vi "motor.vi"() -> ()   [LabVIEW 2020]
uses:
  <vilib>/High Genius/HG_WSI_Tookit/Dependencies/Library/CAN/CAN.lvclass
  C:/Program Files (x86)/National Instruments/LabVIEW 2020/vi.lib/High Genius/HG_WSI_Tookit/Dependencies/Library/HG_LIB/HG_LIB.lvclass
  <vilib>/Platform/TimedLoop/XDataNode/timing_clust.ctl
  <vilib>/Platform/TimedLoop/XDataNode/nitl_modes.ctl
  <vilib>/Platform/TimedLoop/XDataNode/wakeup.ctl
  <vilib>/platform/TimedLoop/XDataNode/XDataNode.xnode
  <vilib>/High Genius/HG_WSI_Tookit/Dependencies/Library/HG_LIB/HG_LIB.lvclass
  <vilib>/Platform/TimedLoop/XDataNode/XDNodeRunTimeDep.lvlib
panel:
  in  "stop":bool
  in  "Numeric":dbl
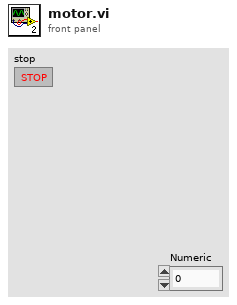
[diagram p1: front panel]
types:
  T1 = enum16{"DI", "DO", "AI", "Pulse", "PWM", "ISQ", "ENC", "CAN", "IIC", "IMU"}
  T2 = enum16{"0", "1", "2", "3", "4", "5", "6", "7", "8", "9", "10", "11", "12", "13", "14", "15", "16", "17", "18", "19", "20", "21", "22", "23", "24", "25"}
  T3 = typedef "XDNodeRunTimeDep.lvlib/timing_clust.ctl" = cluster{"Expected End [f-1]":u64, "Actual End [f-1]":u64, "Finished Late? [f-1]":bool, "Expected End [i-1]":u64, "Actual End [i-1]":u64, "Finished Late? [i-1]":bool, "Expected Start [i]":u64, "Actual Start [i]":u64, "Expected Start [f]":u64, "Actual Start [f]":u64, "Source Name":string, "Structure Name":string, "Period":i64, "Deadline":i64, "Offset":i64, "Start":i64, "Priority":i32, "Timeout":i32, "Mode":T4, "Wakeup Reason":T5, "Error":errorcluster, "Source Type":string, "Secondary Source Type":string, "Global End Time":u64, "Global Start Time":u64, "Frame Duration":u64, "Iteration Duration":u64, "Assigned CPU":i32, "I/O Scan Engine Mode":u32}
  T4 = typedef "XDNodeRunTimeDep.lvlib/nitl_modes.ctl" = enum32{"No Change", "Process missed periods, maintain original phase", "Discard missed periods, maintain original phase", "Process missed periods, ignore original phase", "Discard missed periods, ignore original phase"}
  T5 = typedef "XDNodeRunTimeDep.lvlib/wakeup.ctl" = enum32{"Normal", "Aborted", "Asynchronous wakeup", "Timing source error", "Timed loop error", "Timeout"}
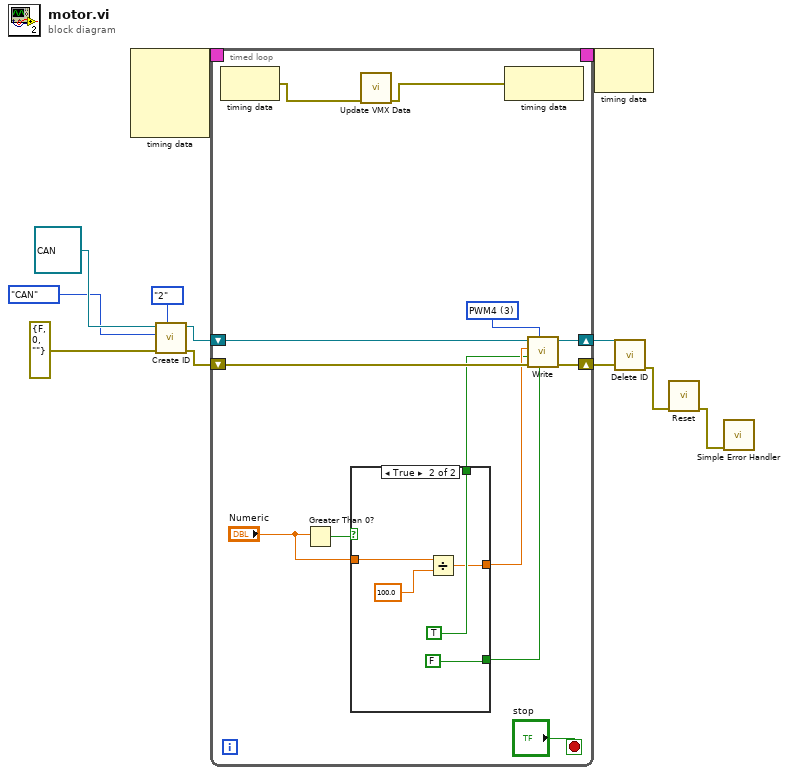
[diagram p0: block diagram]
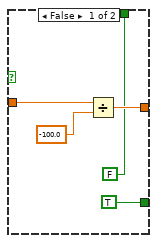
[diagram p2: hidden frame]
diagram:
  n1 = node-c288() -> (w12:T3)  [unwired: 4 in]
  n2 = call <vilib>:"Create ID.vi"("NO"=T2."2", "error in (no error)"=errorcluster {"status"=FALSE, "code"=0, "source"=""}, "Function"=T1."CAN", "HG_LIB in"=refnum<class "CAN.lvclass"> refnum ("VMX Library.lvlib:CAN.lvclass")) -> ("error out"=w4:errorcluster, "HG_LIB out"=w6:refnum<class "CAN.lvclass">)  [unwired: 6 in]
  n3 = timed-loop {
    timing: w12 -> [_]
    timing-out: [_] -> w11
    shift-right: [w22] -> w5
    shift-left: w6 -> [w23]
    shift-right: [w20] -> w3
    shift-left: w4 -> [w21]
    stop <- "stop" stop-if-true
    w14 = u16 3 items=["PWM1", "PWM2", "PWM3", "PWM4"] ("PWM")
    n4 = node-c288() -> (w25:errorcluster)  [unwired: 1 in]
    n5 = Greater Than 0?(x="Numeric") -> (x > 0?=w19:bool)
    n6 = case shown="True" w19 {
      tunnel: "Numeric" -> [w30 w32]
      tunnel: [w28 w31] -> w17
      tunnel: [FALSE TRUE] -> w16
      tunnel: [TRUE FALSE] -> w15
      frame False {
        n7 = Divide(x=w30, y=-100.0) -> (x/y=w28:dbl)
      }
      frame True {
        n8 = Divide(x=w32, y=100.0) -> (x/y=w31:dbl)
      }
    }
    n9 = call <vilib>:"Update VMX Data.vi"("error in (no error)"=w25) -> ("error out"=w24:errorcluster)  [unwired: 10 in]
    n10 = node-c288(w24) -> ()  [unwired: 1 out]
    n11 = call <vilib>:"Write.vi"("INB"=w15, "PWM"=w14, "error in (no error)"=w21, "INA"=w16, "Duty Cycle"=w17, "CAN in"=w23) -> ("error out"=w20:errorcluster, "CAN out"=w22:refnum<class "CAN.lvclass">)  [unwired: 4 in]
  }
  n12 = node-c288(w11) -> ()  [unwired: 1 out]
  n13 = call <vilib>:"Delete ID.vi"("error in (no error)"=w3, "HG_LIB in"=w5) -> ("error out"=w2:errorcluster)  [unwired: 8 in, 1 out]
  n14 = call <vilib>:"Reset.vi"("error in (no error)"=w2) -> ("error out"=w1:errorcluster)  [unwired: 10 in]
  n15 = call <vilib>:"Simple Error Handler.vi"("error in (no error)"=w1) -> ()  [unwired: 4 in, 5 out]
